vi "Enable Auth.vi"(6 "Role Hierarchy (None)":T1[](array[typedef]), 7 "Optional Providers (Basic)":T2, 8 "error in (no error)":errorcluster, 9 "Auth Handlers (Built-In)":T3, 10 "User Provider":refnum<class "User Provider.lvclass">, 11 "Server in":refnum<class "Server.lvclass">) -> (0 "error out":errorcluster, 3 "Server out":refnum<class "Server.lvclass">)   [LabVIEW 2020, in "HTTP Server.lvlib" / "Server.lvclass"]
doc: "Enables automated authentication capabilities by minimally specifying a User Provider implementation and optionally overriding every aspect about how logins, automatic login redirects, authentication errors, authentication and authorization, and user storage and retrieval works.\n\nThe default password encoder uses salting and hashing to secure passwords in a single-direction operation. The password is dual-salted and hashed with SHA256 with the result Base64 encoded.\n\nThe rest of the default handlers are implemented around form authentication and utilize sessions to persist users across requests. Other mechanisms can be implemented such as API keys or bearer tokens embedded as headers that must be supplied with every request. It is also possible to implement authentication mechanisms that tie into other auth mechanisms such as OAuth, Microsoft IAM, etc."
uses:
  Server.lvclass
  Auth Handlers.ctl
  Request Handler/Request Handler.lvclass
  Response Handler/Response Handler.lvclass
  Exception Handler/Exception Handler.lvclass
  Optional Providers.ctl
  Password Encoder/Password Encoder.lvclass
  C:/dev/lv20CE/relink/lv-http-server/HTTP Server/Service/Service.lvclass
  Authentication Provider/Authentication Provider.lvclass
  User Provider/User Provider.lvclass
  Role Inheritance.ctl
  Authentication Handler/Authentication Handler.lvclass
  C:/dev/lv20CE/relink/lv-http-server/HTTP Server/Exception Handler/Exception Handler.lvclass
  C:/dev/lv20CE/relink/lv-http-server/HTTP Server/Response Handler/Response Handler.lvclass
  C:/dev/lv20CE/relink/lv-http-server/HTTP Server/Request Handler/Request Handler.lvclass
  BasicPasswordEncoder/BasicPasswordEncoder.lvclass
  C:/dev/lv20CE/relink/lv-http-server/HTTP Server/Password Encoder/Password Encoder.lvclass
  FormAuthentication/FormAuthentication.lvclass
  C:/dev/lv20CE/relink/lv-http-server/HTTP Server/Authentication Provider/Authentication Provider.lvclass
  Security/Security.lvclass
  Server.lvclass/Server.ctl
  HTTP Server.lvlib
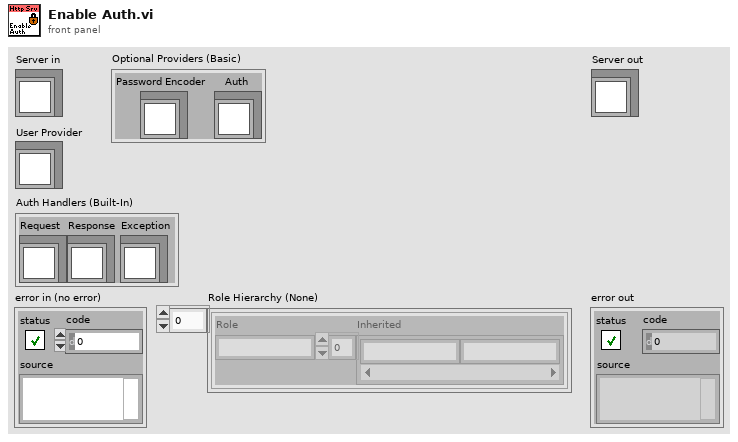
[diagram p1: front panel]
types:
  T1 = typedef "HTTP Server.lvlib/Role Inheritance.ctl" = cluster{"Role":string, "Inherited":string[]}
  T2 = typedef "HTTP Server.lvlib/Optional Providers.ctl" = cluster{"Password Encoder":refnum<class "Password Encoder.lvclass">, "Auth":refnum<class "Authentication Provider.lvclass">}
  T3 = typedef "HTTP Server.lvlib/Auth Handlers.ctl" = cluster{"Request":refnum<class "Request Handler.lvclass">, "Response":refnum<class "Response Handler.lvclass">, "Exception":refnum<class "Exception Handler.lvclass">}
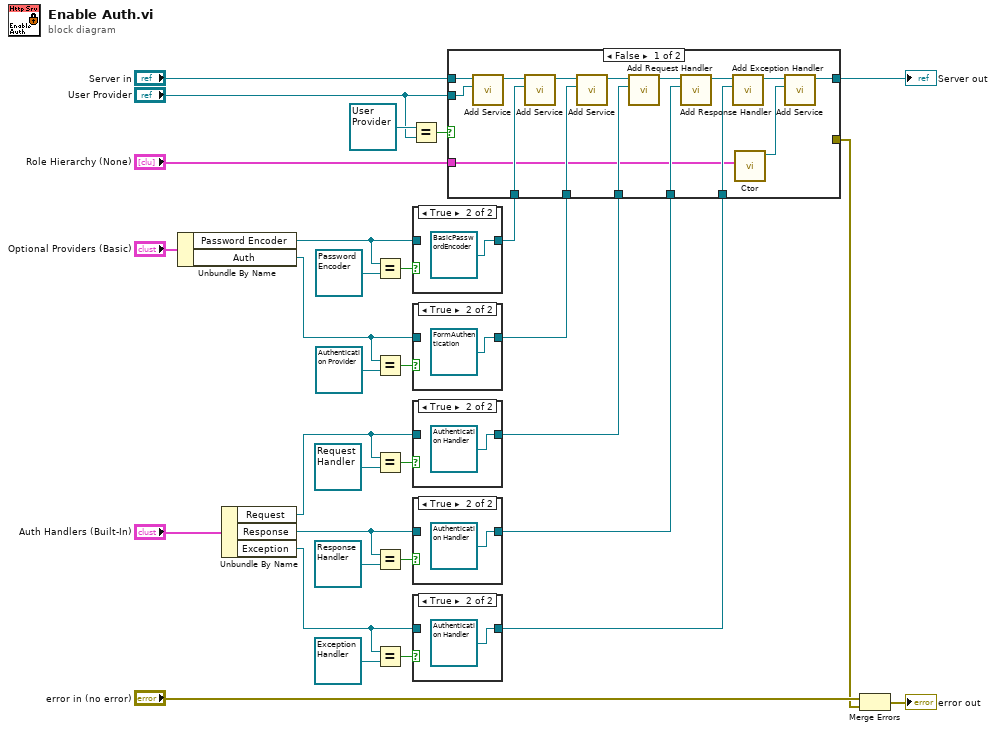
[diagram p0: block diagram]
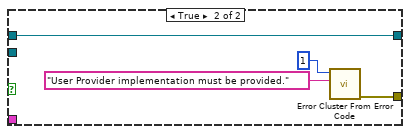
[diagram p7: hidden frame]
diagram:
  n1 = Unbundle By Name("Optional Providers (Basic)") -> ("Password Encoder"=w8:refnum<class "Password Encoder.lvclass">, "Auth"=w7:refnum<class "Authentication Provider.lvclass">)
  n2 = Unbundle By Name("Auth Handlers (Built-In)") -> ("Request"=w10:refnum<class "Request Handler.lvclass">, "Response"=w12:refnum<class "Response Handler.lvclass">, "Exception"=w11:refnum<class "Exception Handler.lvclass">)
  n3 = Equal?(x=w8, y=refnum<class "Password Encoder.lvclass"> refnum) -> (x = y?=w28:bool)
  n4 = Equal?(x=w7, y=refnum<class "Authentication Provider.lvclass"> refnum ("Auth Provider (Default Form)")) -> (x = y?=w29:bool)
  n5 = Equal?(x=w10, y=refnum<class "Request Handler.lvclass"> refnum) -> (x = y?=w25:bool)
  n6 = Equal?(x=w12, y=refnum<class "Response Handler.lvclass"> refnum) -> (x = y?=w23:bool)
  n7 = Equal?(x=w11, y=refnum<class "Exception Handler.lvclass"> refnum) -> (x = y?=w22:bool)
  n8 = Equal?(x=refnum<class "User Provider.lvclass"> refnum, y="User Provider") -> (x = y?=w5:bool)
  n9 = case shown="True" w28 {
    tunnel: w8 -> [w32 _]
    tunnel: [w32 refnum<class "BasicPasswordEncoder.lvclass"> refnum ("HTTP Server.lvlib:BasicPasswordEncoder.lvclass")] -> w16
    frame False {
    }
    frame True {
    }
  }
  n10 = case shown="True" w29 {
    tunnel: w7 -> [w34 _]
    tunnel: [w34 refnum<class "FormAuthentication.lvclass"> refnum ("HTTP Server.lvlib:FormAuthentication.lvclass")] -> w15
    frame False {
    }
    frame True {
    }
  }
  n11 = case shown="True" w25 {
    tunnel: w10 -> [w36 _]
    tunnel: [w36 refnum<class "Authentication Handler.lvclass"> refnum ("HTTP Server.lvlib:Authentication Handler.lvclass")] -> w24
    frame False {
    }
    frame True {
    }
  }
  n12 = case shown="True" w23 {
    tunnel: w12 -> [w38 _]
    tunnel: [w38 refnum<class "Authentication Handler.lvclass"> refnum ("HTTP Server.lvlib:Authentication Handler.lvclass")] -> w19
    frame False {
    }
    frame True {
    }
  }
  n13 = case shown="True" w22 {
    tunnel: w11 -> [w40 _]
    tunnel: [w40 refnum<class "Authentication Handler.lvclass"> refnum ("HTTP Server.lvlib:Authentication Handler.lvclass")] -> w18
    frame False {
    }
    frame True {
    }
  }
  n14 = case shown="False" w5 {
    tunnel: w24 -> [w57 _]
    tunnel: w19 -> [w54 _]
    tunnel: w18 -> [w53 _]
    tunnel: "Server in" -> [w52 w61]
    tunnel: w16 -> [w51 _]
    tunnel: w15 -> [w48 _]
    tunnel: [w44 w61] -> w14
    tunnel: "User Provider" -> [w43 _]
    tunnel: [_ w58] -> w3
    tunnel: "Role Hierarchy (None)" -> [w42 _]
    frame False {
      n15 = call "Add Service.vi"("Service"=w43, "Server in"=w52) -> ("Server out"=w50:refnum<class "Server.lvclass">)  [unwired: 8 in, 1 out]
      n16 = call "Add Service.vi"("Service"=w51, "Server in"=w50) -> ("Server out"=w49:refnum<class "Server.lvclass">)  [unwired: 8 in, 1 out]
      n17 = call "Add Service.vi"("Service"=w48, "Server in"=w49) -> ("Server out"=w47:refnum<class "Server.lvclass">)  [unwired: 8 in, 1 out]
      n18 = call "Add Request Handler.vi"("Request Handler"=w57, "Server in"=w47) -> ("Server out"=w56:refnum<class "Server.lvclass">)  [unwired: 8 in, 1 out]
      n19 = call "Add Response Handler.vi"("Response Handler"=w54, "Server in"=w56) -> ("Server out"=w55:refnum<class "Server.lvclass">)  [unwired: 8 in, 1 out]
      n20 = call "Add Exception Handler.vi"("Exception Handler"=w53, "Server in"=w55) -> ("Server out"=w46:refnum<class "Server.lvclass">)  [unwired: 8 in, 1 out]
      n21 = call "Ctor.vi"("Role Hierarchy (None)"=w42) -> ("Security out"=w45:refnum<class "Security.lvclass">)  [unwired: 9 in, 1 out]
      n22 = call "Add Service.vi"("Service"=w45, "Server in"=w46) -> ("Server out"=w44:refnum<class "Server.lvclass">)  [unwired: 8 in, 1 out]
    }
    frame True {
      n23 = call <vilib>:"Error Cluster From Error Code.vi"("error message (\"\")"="User Provider implementation must be provided." ("error message (\"\")"), "error code (0)"=1) -> ("error out"=w58:errorcluster)  [unwired: 7 in]
    }
  }
  "Server out" <- w14
  n24 = Merge Errors("error in (no error)", w3) -> (→"error out":errorcluster)
